vi "Wavepond Test Harness.vi"   [LabVIEW 2014, in "Wavepond.lvclass"]
uses:
  Wavepond.lvclass
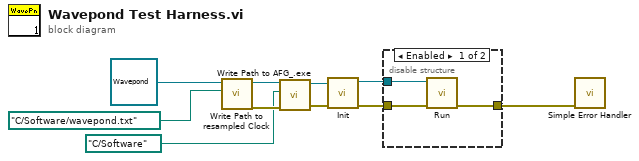
[diagram p0: block diagram]
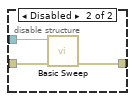
[diagram p2: hidden frame]
diagram:
  n1 = call-dynamic "Write Path to resampled Clock.vi"("Path to resampled Clock"=path "C:/Software/wavepond.txt", "Wavepond in"=refnum<class "Wavepond.lvclass"> refnum ("Wavepond.lvclass")) -> ("error out"=w8:errorcluster, "Wavepond out"=w7:refnum<class "Wavepond.lvclass">)  [unwired: 8 in]
  n2 = call-dynamic "Write Path to AFG_.exe.vi"("error in (no error)"=w8, "Path to AFG*.exe"=path "C:/Software" ("Path to resampled Clock"), "Wavepond in"=w7) -> ("error out"=w5:errorcluster, "Wavepond out"=w6:refnum<class "Wavepond.lvclass">)  [unwired: 7 in]
  n3 = call-dynamic "Init.vi"("error in (no error)"=w5, "DtoA in"=w6) -> ("error out"=w2:errorcluster, "DtoA out"=w1:refnum<class "Wavepond.lvclass">)  [unwired: 8 in]
  n4 = disable-structure shown="Enabled" {
    disable-tunnel: [w13 w14] -> w3
    disable-tunnel: w2 -> [w12 w15]
    disable-tunnel: w1 -> [w11 w16]
    frame Enabled {
      n5 = call-dynamic "Run.vi"("error in (no error)"=w12, "Wavepond in"=w11) -> ("error out"=w13:errorcluster)  [unwired: 8 in, 1 out]
    }
    frame Disabled {
      n6 = call-dynamic "Basic Sweep.vi"("error in (no error)"=w15, "Wavepond in"=w16) -> ("error out"=w14:errorcluster)  [unwired: 8 in, 1 out]
    }
  }
  n7 = call <vilib>:"Simple Error Handler.vi"("error in (no error)"=w3) -> ()  [unwired: 4 in, 5 out]
